vi "get_component_type_name.vi"(8 "error in (no error)":errorcluster, 11 "GenericStringGenerator in":refnum<class "GenericStringGenerator.lvclass">) -> (0 "error out":errorcluster, 2 "component type":string, 3 "GenericStringGenerator out":refnum<class "GenericStringGenerator.lvclass">)   [LabVIEW 2010, in "GenericStringGenerator.lvclass"]
uses:
  GenericStringGenerator.lvclass
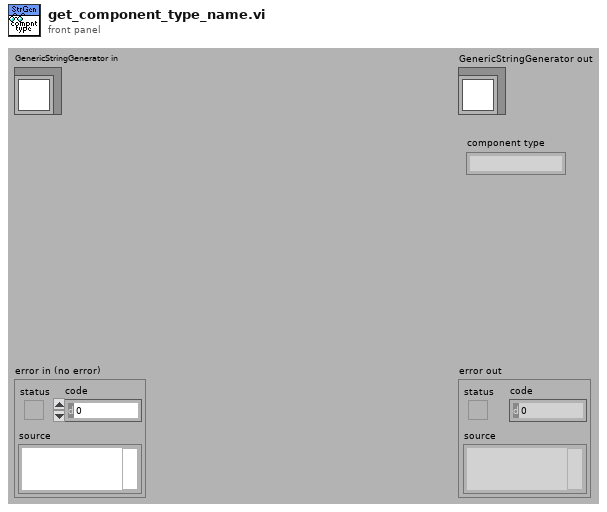
[diagram p1: front panel]
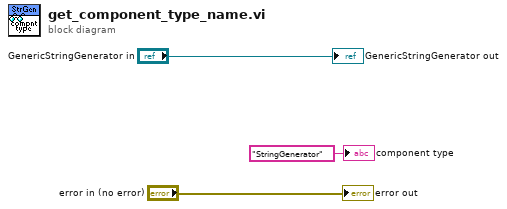
[diagram p0: block diagram]
diagram:
  "error out" <- "error in (no error)"
  "GenericStringGenerator out" <- "GenericStringGenerator in"
  "component type" <- "StringGenerator" ("component type")
